vi "GetPID.vi"(8 "error in (no error)":errorcluster) -> (0 "error out":errorcluster, 2 "return type":i32)   [LabVIEW 2014]
uses:
  Kernel32.dll
panel:
  # "This VI should be called on running LabVIEW \nand not nilvcli.dll context."
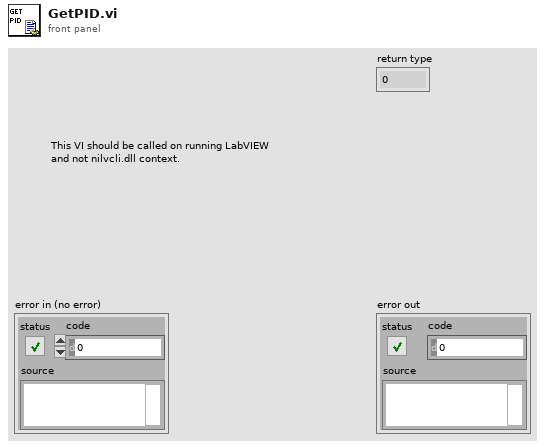
[diagram p1: front panel]
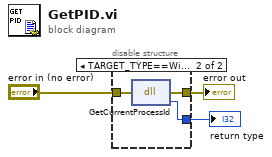
[diagram p0: block diagram]
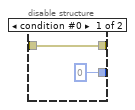
[diagram p2: hidden frame]
diagram:
  n1 = disable-structure shown="TARGET_TYPE==Windows" {
    disable-tunnel: "error in (no error)" -> [w4 w8]
    disable-tunnel: [0 ("return type 2") w7] -> w2
    disable-tunnel: [w4 w6] -> w1
    frame condition #0 {
    }
    frame condition #1 (active) {
      n2 = dll-call lib="Kernel32.dll" fn="GetCurrentProcessId"(error in=w8) -> (error out=w6:errorcluster, "return type"=w7:i32)  [unwired: 2 in, 1 out]
    }
  }
  "return type" <- w2
  "error out" <- w1
